vi "Get Frame Port Reference.vi"(8 "error in":errorcluster, 11 "Frame Ref":T1 format="%.0x") -> (0 "error out":errorcluster, 3 "Port Ref":T1 format="%.0x")   [LabVIEW 2020, in "Communication Bus Template Scripting.lvlib"]
uses:
  Communication Bus Template Scripting.lvlib
  <vilib>/NI VeriStand/Custom Device API/Custom Device Item Ref.ctl
  <vilib>/NI VeriStand/Custom Device Tools/Custom Device Utility Library/Search Direction.ctl
  System Explorer/Constants.vi
  <vilib>/NI VeriStand/Custom Device Tools/Custom Device Utility Library/NI VeriStand - Search for Item by GUID.vi
  <vilib>/NI VeriStand/Custom Device Tools/Custom Device Utility Library/Custom Device Utility Library.lvlib
  <vilib>/NI VeriStand/Custom Device API/Custom Device API.lvlib
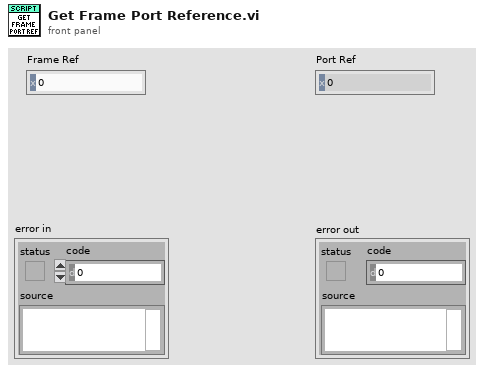
[diagram p1: front panel]
types:
  T1 = typedef "Custom Device API.lvlib/Custom Device Item Ref.ctl" = u64
  T2 = typedef "Custom Device Utility Library.lvlib/Search Direction.ctl" = enum16{"Down", "Up"}
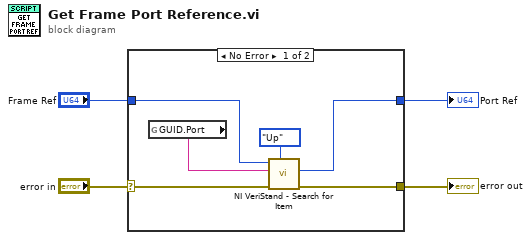
[diagram p0: block diagram]
diagram:
  n1 = case shown="No Error" "error in" {
    selector: "error in" -> [w9 w11]
    tunnel: [w8 w11] -> w3
    tunnel: "Frame Ref" -> [w7 _]
    tunnel: [w6 _] -> w1
    frame No Error {
      n2 = global read "Constants.vi" "GUID.Port"() -> (w5:string)
      n3 = call-poly <vilib>:"NI VeriStand - Search for Item.vi"("Direction (Down)"=Search_Direction."Up", "error in"=w9, "Item GUID"=w5, "Section Ref in"=w7) -> ("error out"=w8:errorcluster, "Item Ref"=w6:T1)  [unwired: 4 in, 2 out]
    }
    frame Error {
    }
  }
  "Port Ref" <- w1
  "error out" <- w3
